vi "RequiredForInterface-ActionDefs.vi"(8 "error in (no error)":errorcluster, 11 "Class-Interface in":refnum<class "Class-Interface.lvclass">) -> (0 "error out":errorcluster, 2 "Configuration List":T1[](array[typedef])=[{"Name"="OpenDevice", "ConfigurationPrototype"=variant(cluster{"DeviceType":string, "DeviceIndex":u32} {"DeviceType"="", "DeviceIndex"=0}), "ResultPrototype"=variant}, {"Name"="TransmitData", "ConfigurationPrototype"=variant(cluster{"Channel Num":u32, "Frame":cluster{"Identifier":u32, "PayLoad":cluster{"byte1":u8, "byte2":u8, "byte3":u8, "byte4":u8, "byte5":u8, "byte6":u8, "byte7":u8, "byte8":u8}}} {"Channel Num"=0, "Frame"={"Identifier"=0, "PayLoad"={"byte1"=0, "byte2"=0, "byte3"=0, "byte4"=0, "byte5"=0, "byte6"=0, "byte7"=0, "byte8"=0}}}), "ResultPrototype"=variant}, {"Name"="ReceiveData", "ConfigurationPrototype"=variant(cluster{"Channel Num":u32, "timeout(ms)":i32} {"Channel Num"=0, "timeout(ms)"=50}), "ResultPrototype"=variant(cluster{"Identifier":u32, "PayLoad":u8[]} {"Identifier"=0, "PayLoad"=[]})}, {"Name"="CloseDevice", "ConfigurationPrototype"=variant, "ResultPrototype"=variant}, {"Name"="InitCAN", "ConfigurationPrototype"=variant(cluster{"Channel Num":u32} {"Channel Num"=0}), "ResultPrototype"=variant}, {"Name"="Config-BaudRate", "ConfigurationPrototype"=variant(cluster{"Channel Num":u32, "BaudRate":u32} {"Channel Num"=0, "BaudRate"=125000}), "ResultPrototype"=variant}, {"Name"="Config-Termination", "ConfigurationPrototype"=variant(cluster{"Channel Num":u32, "Termination":enum8{"on", "off"}} {"Channel Num"=0, "Termination"=enum."on"}), "ResultPrototype"=variant}] caption="Value auto generated by TOOLs", 3 "Class-Interface out":refnum<class "Class-Interface.lvclass">)   [LabVIEW 2019, in "CAN-Interface.lvlib" / "Class-Interface.lvclass"]
uses:
  Class-Interface.lvclass
  <vilib>/LVAPT/.lib/HAL-Interface.lvlibp/HALInterface/Typedef/Def-ActionPrototype.ctl
  <vilib>/LVAPT/.lib/HAL-Interface.lvlibp/HALInterface/HALInterface.lvclass
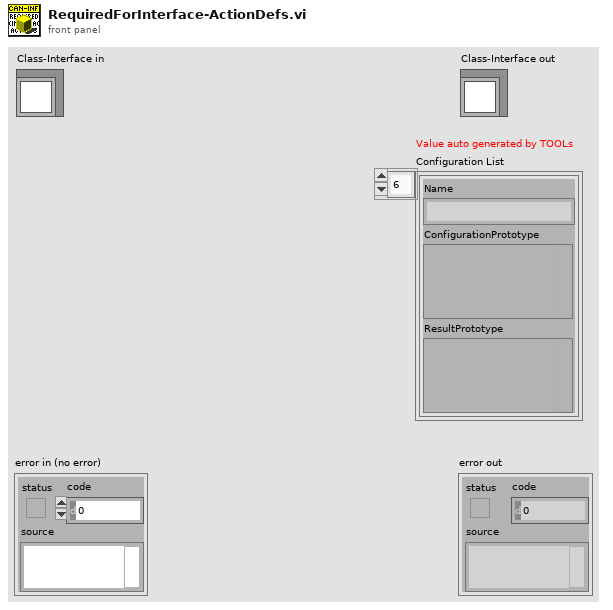
[diagram p1: front panel]
types:
  T1 = typedef "HAL-Interface.lvlibp/HALInterface.lvclass/Def-ActionPrototype.ctl" = cluster{"Name":string, "ConfigurationPrototype":variant, "ResultPrototype":variant}
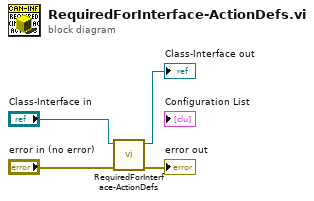
[diagram p0: block diagram]
diagram:
  n1 = call-parent "RequiredForInterface-ActionDefs.vi"("error in (no error)"="error in (no error)", "HALInterface in"="Class-Interface in") -> ("error out"=→"error out":errorcluster, "HALInterface out"=→"Class-Interface out":refnum<class "Class-Interface.lvclass">)  [unwired: 7 in, 1 out]
